vi "Initialize Output DMA Refs.vi"(8 "error in (no error)":errorcluster, 10 "Settings.Compiled":T1 {"IncomingRegisters.Settings"."Register"."Data Type" format="%.0x"; "IncomingRegisters.Refs"."Refs"."Data Reference" format="%.0x"; "OutgoingRegisters.Settings"."Register"."Data Type" format="%.0x"; "OutgoingRegisters.Refs"."Refs"."Data Reference" format="%.0x"; "IncomingDMA.Settings"."DMA.Settings"."DMA Host Buffer" items=["1 Second"=1, "2 Seconds"=2, "5 Seconds"=5, "10 Seconds"=10]; "IncomingDMA.Settings"."DMA.Settings"."dt" format="%#_p"; "IncomingDMA.Settings"."DMA.Settings"."Update Rate" items=["1 Hz"=1, "2 Hz"=2, "5 Hz"=5, "10 Hz"=10]; "OutgoingDMA.Settings"."DMA.Settings"."DMA Host Buffer" items=["1 Second"=1, "2 Seconds"=2, "5 Seconds"=5, "10 Seconds"=10]; "OutgoingDMA.Settings"."DMA.Settings"."dt" format="%#_p"; "OutgoingDMA.Settings"."DMA.Settings"."Update Rate" items=["1 Hz"=1, "2 Hz"=2, "5 Hz"=5, "10 Hz"=10]}, 11 "FPGA Ref":refnum<k20>) -> (0 "error out":errorcluster, 2 "DMA":T15[](array[typedef]), 3 "FPGA Ref":refnum<k20>)   [LabVIEW 2016, in "FPGA Addon Engine.lvlib"]
uses:
  FPGA Addon Engine.lvlib
  Types/DMA Output References.ctl
  <vilib>/NI Veristand/Custom Device Waveform API/Single Waveform Read (DBL)/Single Waveform Read (DBL).lvclass
  Types/DMA Output Ref.ctl
  Shared/Compiled.Settings.ctl
  Shared/Compiled.RegisterSettings.ctl
  Shared/Scalar Type.ctl
  Shared/Register Information.ctl
  Shared/Data Type.ctl
  <vilib>/NI Veristand/Custom Device API/Block Data Reference.ctl
  <vilib>/NI Veristand/Custom Device API/Data Reference.ctl
  Shared/Compiled.DMASettings.ctl
  Shared/DMA Settings.ctl
  Shared/Delacing Scheme.ctl
  Shared/DMA Acquisition Mode.ctl
  <vilib>/NI Veristand/Custom Device API/Waveform Data Reference.ctl
  Shared/FPGA Settings.ctl
  <vilib>/NI Veristand/Custom Device API/Custom Device Target Type.ctl
  <vilib>/NI/LVFPGA Adv Session Resources/OpenByNameSubVI.vi
  <vilib>/NI Veristand/Custom Device Waveform API/Single Waveform Read (DBL)/NI VeriStand - Open Single Waveform Read Session (DBL).vi
  <vilib>/Utility/error.llb/Error Cluster From Error Code.vi
  <vilib>/rvi/interface/common/niFpgaWaitOnOcc.vi
  <vilib>/rvi/interface/common/dynamic/niFpgaEscapeDelimiterAndNull.vi
  <vilib>/rvi/interface/nirviMethod/nirviMethod.xnode
  <vilib>/NI/LVFPGA Adv Session Resources/OpenByName.xnode
  <vilib>/NI VeriStand/Custom Device Waveform API/NI_VS Custom Device Waveform API.lvlib
  <vilib>/rvi/errors/niLvFpgaMergeErrorWithErrorCode.vi
  <vilib>/FPGAPlugInAG/Dynamic/niLvFpga_ConfigureFifo_Dynamic.vi
  <vilib>/FPGAPlugInAG/Dynamic/niLvFpga_StartFifo_Dynamic.vi
  <vilib>/NI/LVFPGA Adv Session Resources/LVFPGAAdvSessionResources.lvlib
  <vilib>/NI VeriStand/Custom Device API/Custom Device API.lvlib
  Shared/FPGA Addon Shared.lvlib
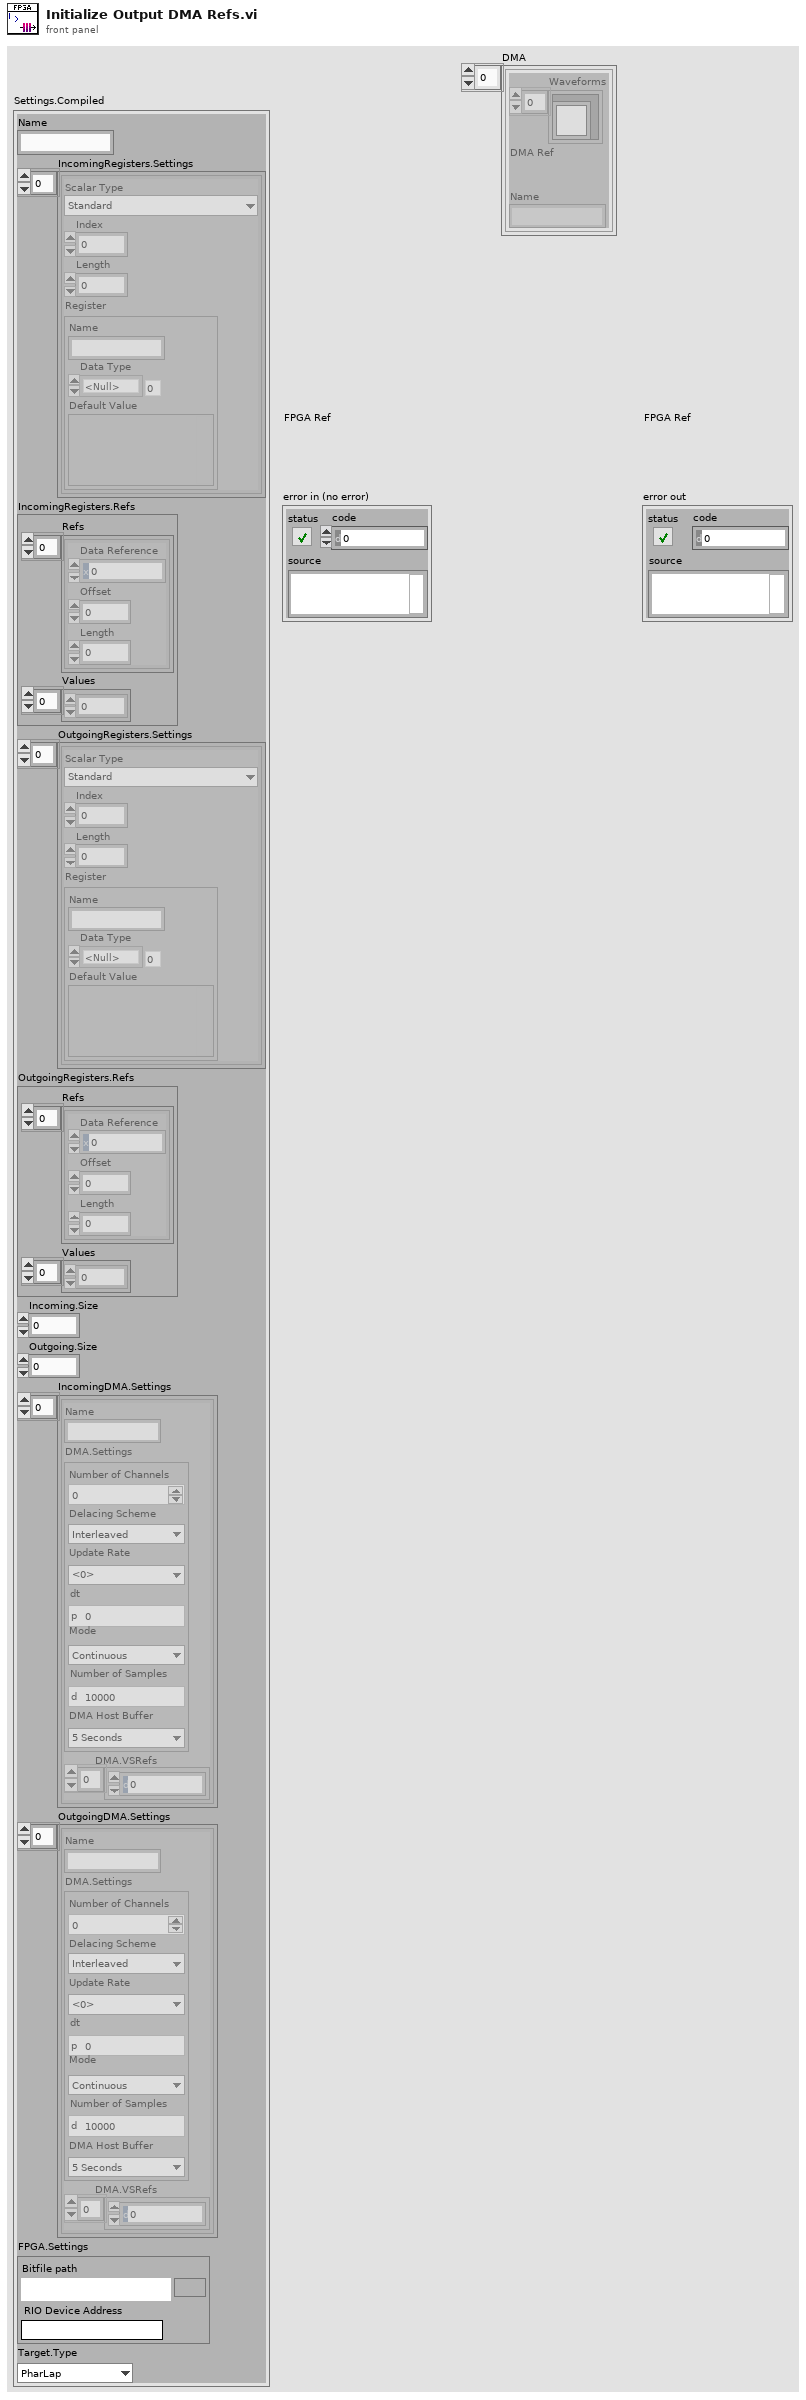
[diagram p1: front panel]
types:
  T1 = typedef "FPGA Addon Shared.lvlib/Compiled.Settings.ctl" = cluster{"Name":string, "IncomingRegisters.Settings":T2[], "IncomingRegisters.Refs":cluster{"Refs":T6[], "Values":dbl[]}, "OutgoingRegisters.Settings":T2[], "OutgoingRegisters.Refs":cluster{"Refs":T6[], "Values":dbl[]}, "Incoming.Size":i32, "Outgoing.Size":i32, "IncomingDMA.Settings":T8[], "OutgoingDMA.Settings":T8[], "FPGA.Settings":T13, "Target.Type":T14}
  T2 = typedef "FPGA Addon Shared.lvlib/Compiled.RegisterSettings.ctl" = cluster{"Scalar Type":T3, "Index":i32, "Length":i32, "Register":T4}
  T3 = typedef "FPGA Addon Shared.lvlib/Scalar Type.ctl" = enum16{"Standard", "Bitpacked"}
  T4 = typedef "FPGA Addon Shared.lvlib/Register Information.ctl" = cluster{"Name":string, "Data Type":T5, "Default Value":variant}
  T5 = typedef "FPGA Addon Shared.lvlib/Data Type.ctl" = enum8{"<Null>", "I8", "I16", "I32", "I64", "U8", "U16", "U32", "U64", "SGL", "Boolean", "Analog PWM In Settings", "Analog PWM In", "Digital PWM In Settings", "Digital PWM In", "Digital PWM Out", "Sine Out", "FXP+/-24.5", "FXP+/-16.5", "FXP+/-32.8", "FXP+/-64.32", "FXP+/-16.7", "FXP+/-20.5"}
  T6 = typedef "Custom Device API.lvlib/Block Data Reference.ctl" = cluster{"Data Reference":T7, "Offset":u64, "Length":u64}
  T7 = typedef "Custom Device API.lvlib/Data Reference.ctl" = i32
  T8 = typedef "FPGA Addon Shared.lvlib/Compiled.DMASettings.ctl" = cluster{"Name":string, "DMA.Settings":T9, "DMA.VSRefs":T12[]}
  T9 = typedef "FPGA Addon Shared.lvlib/DMA Settings.ctl" = cluster{"Number of Channels":u8, "Delacing Scheme":T10, "Update Rate":u32, "dt":dbl, "Mode":T11, "Number of Samples":u32, "DMA Host Buffer":u32}
  T10 = typedef "FPGA Addon Shared.lvlib/Delacing Scheme.ctl" = enum8{"Interleaved"}
  T11 = typedef "FPGA Addon Shared.lvlib/DMA Acquisition Mode.ctl" = enum8{"Continuous", "Triggered Finite"}
  T12 = typedef "Custom Device API.lvlib/Waveform Data Reference.ctl" = i32
  T13 = typedef "FPGA Addon Shared.lvlib/FPGA Settings.ctl" = cluster{"Bitfile path":path, "RIO Device Address":string}
  T14 = typedef "Custom Device API.lvlib/Custom Device Target Type.ctl" = enum16{"PharLap", "VxWorks", "Windows", "Linux_32_ARM", "Linux_x64"}
  T15 = typedef "FPGA Addon Engine.lvlib/DMA Output References.ctl" = cluster{"Waveforms":refnum<class "Single Waveform Read (DBL).lvclass">[], "DMA Ref":T16, "Name":string}
  T16 = typedef "FPGA Addon Engine.lvlib/DMA Output Ref.ctl" = refnum<k20>
  T17 = cluster{"Name":string, "Depth":u32, "Write? (Deprecated:Use Implementation)":bool, "Physical Channel":u32, "Base Address":u32, "Data Width":u32, "Data Type":enum32{"Boolean", "I8", "I16", "I32", "I64", "U8", "U16", "U32", "U64", "FXP", "CustomControl", "SGL"}, "FXP Properties":variant, "Write Window Address":u32, "Implementation":enum16{"niFpgaTargetToHost", "niFpgaHostToTarget", "niFpgaPeerToPeerWriter", "niFpgaPeerToPeerReader", "niCoreTargetToHost", "niCoreHostToTarget"}, "Control Set":u32}[]
  T18 = cluster{"Name":string, "type":variant, "indicator?":bool}[]
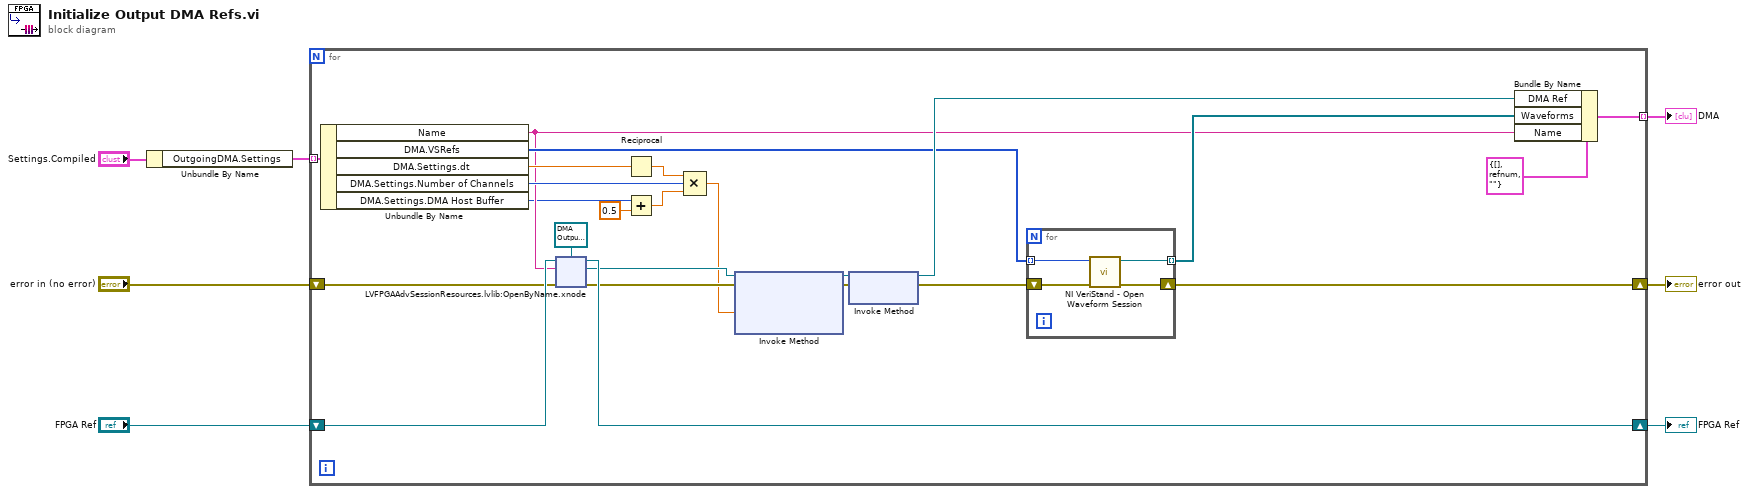
[diagram p0: block diagram]
diagram:
  n1 = Unbundle By Name("Settings.Compiled") -> ("OutgoingDMA.Settings"=w2:T8[])
  n2 = for {
    shift-right: [w12] -> w5
    shift-left: "error in (no error)" -> [w18]
    shift-right: [w29] -> w6
    shift-left: "FPGA Ref" -> [w30]
    tunnel: [w27] -> w4 mode=indexing
    tunnel: w2 -> [w20] mode=indexing
    n3 = Unbundle By Name(w20) -> ("Name"=w14:string, "DMA.VSRefs"=w19:T12[], "DMA.Settings.dt"=w17:dbl, "DMA.Settings.Number of Channels"=w16:u8, "DMA.Settings.DMA Host Buffer"=w10:u32)
    n4 = xnode "LVFPGAAdvSessionResources.lvlib:OpenByName.xnode"("FPGA VI Reference in"=w30, "Resource name in"=w14, "Single resource reference type in"=T16 refnum, "Error in"=w18) -> ("Single resource reference out"=w23:T16, "Error out"=w24:errorcluster, "FPGA VI Reference out"=w29:refnum<k20>)
    n5 = Reciprocal(x=w17) -> (1/x=w11:dbl)
    n6 = Add(x=w10, y=0.5) -> (x+y=w9:dbl)
    n7 = Compound Arithmetic op=MULTIPLY(w11, w16, w9) -> (w21:dbl)
    n8 = xnode "Invoke Method"("FPGA VI Reference In"=w23, "error in"=w24, "Requested Depth"=w21) -> ("FPGA VI Reference Out"=w26:T16, "error out"=w25:errorcluster)  [unwired: 1 out]
    n9 = xnode "Invoke Method"("FPGA VI Reference In"=w26, "error in"=w25) -> ("FPGA VI Reference Out"=w22:T16, "error out"=w13:errorcluster)
    n10 = for {
      shift-right: [w35] -> w12
      shift-left: w13 -> [w33]
      tunnel: [w34] -> w15 mode=indexing
      tunnel: w19 -> [w32] mode=indexing
      n11 = call-poly <vilib>:"NI VeriStand - Open Waveform Session.vi"("error in (no error)"=w33, "DBL Waveform Data Reference"=w32) -> ("error out"=w35:errorcluster, "Single Waveform Read Session (DBL)"=w34:refnum<class "Single Waveform Read (DBL).lvclass">)  [unwired: 8 in]
    }
    n12 = Bundle By Name(cluster=T15 {"Waveforms"=[], "DMA Ref"=refnum, "Name"=""}, "DMA Ref"=w22, "Waveforms"=w15, "Name"=w14) -> (w27:T15)
  }
  "error out" <- w5
  "FPGA Ref" <- w6
  "DMA" <- w4
